vi "Control Servo.vi"(8 "error in (no error)":errorcluster, 9 "setpoint (V)":dbl, 10 "force (V)":dbl, 11 "Controller in":refnum<class "Controller.lvclass">) -> (0 "error out":errorcluster, 2 "servo pw (us)":dbl, 3 "Controller out":refnum<class "Controller.lvclass">)   [LabVIEW 2020, in "Controller.lvclass"]
uses:
  Controller.lvclass
  Controller.lvclass/Controller.ctl
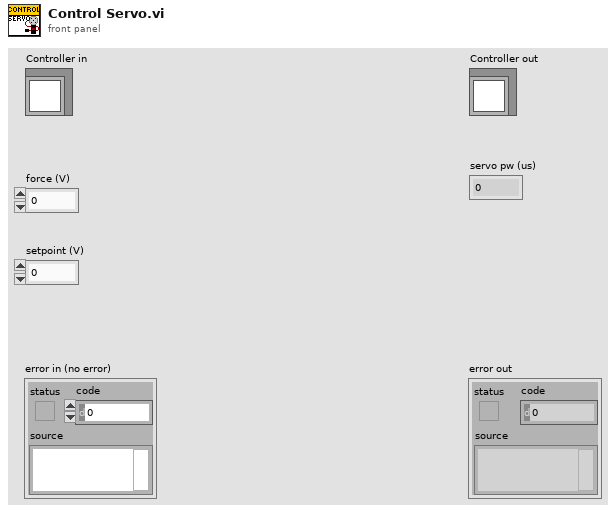
[diagram p1: front panel]
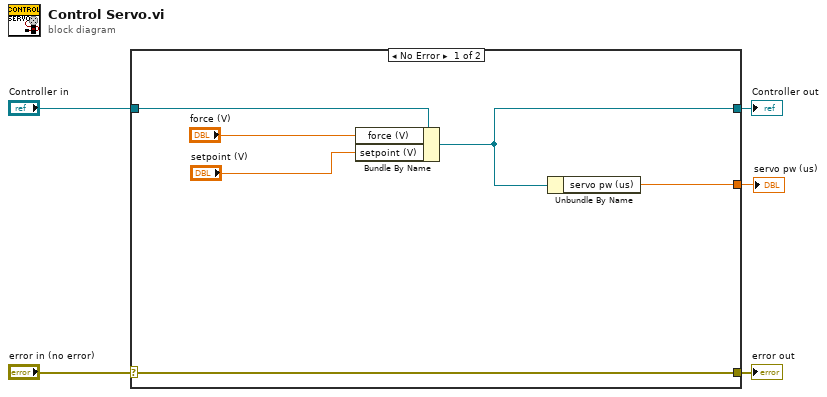
[diagram p0: block diagram]
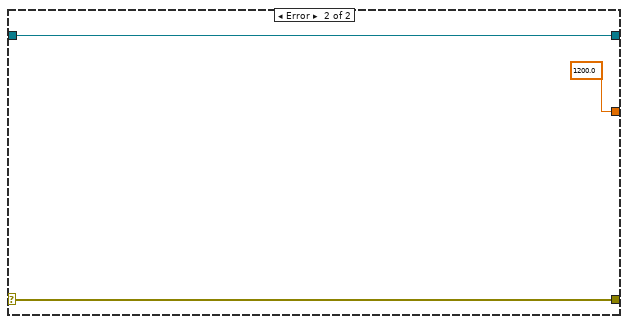
[diagram p2: hidden frame]
diagram:
  n1 = case shown="No Error" "error in (no error)" {
    selector: "error in (no error)" -> [w11 w14]
    tunnel: [w11 w14] -> w4
    tunnel: [w8 w13] -> w2
    tunnel: "Controller in" -> [w9 w13]
    tunnel: [w10 1200.0 ("servo pwm (%)")] -> w1
    frame No Error {
      n2 = Bundle By Name(cluster=w9, "force (V)"="force (V)", "setpoint (V)"="setpoint (V)") -> (w8:refnum<class "Controller.lvclass">)
      n3 = Unbundle By Name(w8) -> ("servo pw (us)"=w10:dbl)
    }
    frame Error {
    }
  }
  "error out" <- w4
  "Controller out" <- w2
  "servo pw (us)" <- w1
